vi "RadiusCheck.vi"(0 "Radius In":dbl) -> (1 "Result":bool, 2 "Radius Out":dbl)   [LabVIEW 2015]
doc: "Check the radius is less than 3. If the radius is less than 3, the result returns true. If the radius is equal or greater than 3, the result return false."
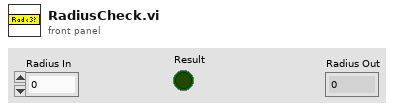
[diagram p1: front panel]
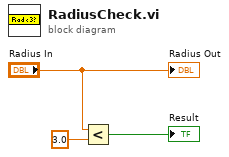
[diagram p0: block diagram]
diagram:
  n1 = Less?(x="Radius In", y=3.0) -> (x < y?=→"Result":bool)
  "Radius Out" <- "Radius In"
